vi "find_special_character_pairs.vi"(8 "error in (no error)":errorcluster, 10 "String Pair":T1={"Start Sting"="{", "End String"="}"}, 11 "Command String":string="TRIGger:AND:ENABle {{ON | 1} | {OFF | 0}}") -> (0 "error out":errorcluster, 2 "Pair Offset":cluster{"Start Offset":i32, "End offset":i32}[](array[cluster])=[{"Start Offset"=21, "End offset"=28}, {"Start Offset"=32, "End offset"=40}, {"Start Offset"=20, "End offset"=41}])   [LabVIEW 2018]
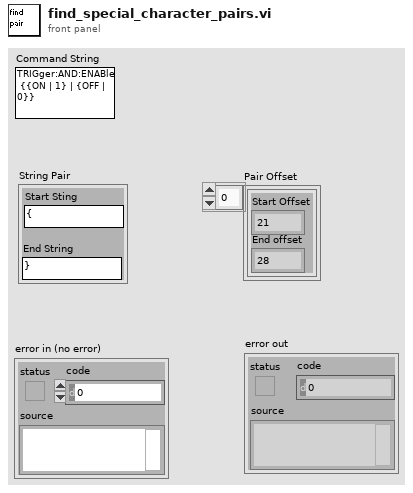
[diagram p1: front panel]
types:
  T1 = cluster{"Start Sting":string, "End String":string}
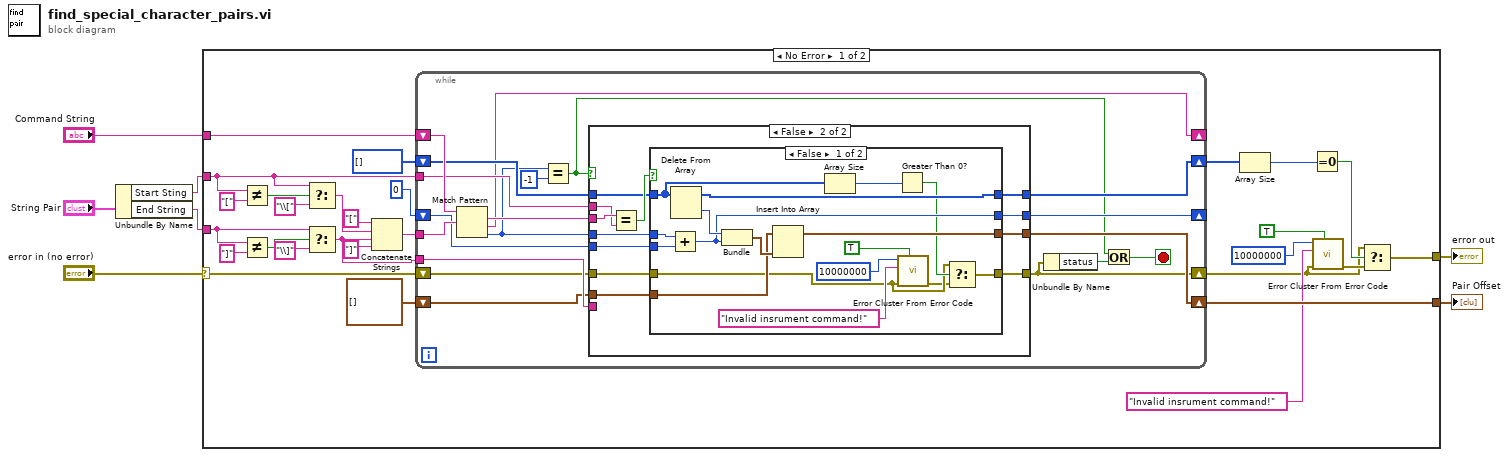
[diagram p0: block diagram]
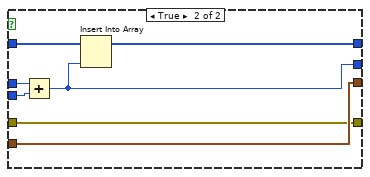
[diagram p3: hidden frame]
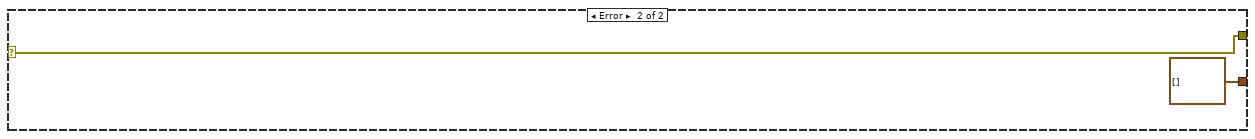
[diagram p4: hidden frame]
diagram:
  n1 = Unbundle By Name("String Pair") -> ("Start Sting"=w2:string, "End String"=w1:string)
  n2 = case shown="No Error" "error in (no error)" {
    selector: "error in (no error)" -> [w27 w96]
    tunnel: "Command String" -> [w33 _]
    tunnel: w1 -> [w10 _]
    tunnel: w2 -> [w8 _]
    tunnel: [w28 cluster{"Start Offset":i32, "End offset":i32}[] [] ("Pair Offset")] -> w6
    tunnel: [w18 w96] -> w4
    frame No Error {
      n3 = Not Equal?(x=w8, y="[") -> (x != y?=w15:bool)
      n4 = Not Equal?(x=w10, y="]") -> (x != y?=w12:bool)
      n5 = Select(t=w8, s=w15, f="\\[") -> (s? t:f=w13:string)
      n6 = Select(t=w10, s=w12, f="\\]") -> (s? t:f=w9:string)
      n7 = Concatenate Strings("[" ("string"), w13, w9, "]" ("string")) -> (w30:string)
      n8 = while {
        shift-right: [w41] -> _
        shift-left: w33 -> [w54]
        shift-right: [w45] -> _
        shift-left: 0 ("y") -> [w46]
        shift-right: [w44] -> w26
        shift-left: i32[] [] -> [w48]
        tunnel: w9 -> [w50]
        tunnel: w8 -> [w51]
        tunnel: w30 -> [w53]
        shift-right: [w42] -> w28
        shift-left: cluster{"Start Offset":i32, "End offset":i32}[] [] ("Pair Offset") -> [w43]
        shift-right: [w36] -> w19
        shift-left: w27 -> [w37]
        stop <- w38 stop-if-true
        n9 = Match Pattern(string=w54, regular expression=w53) -> (match substring=w49:string, after substring=w41:string, offset past match=w47:i32)  [unwired: 2 out]
        n10 = Equal?(x=w47, y=-1) -> (x = y?=w40:bool)
        n11 = case shown="False" w40 {
          tunnel: w51 -> [_ w69]
          tunnel: w50 -> [_ _]
          tunnel: w49 -> [_ w70]
          tunnel: w48 -> [w57 w67]
          tunnel: w47 -> [_ w66]
          tunnel: w46 -> [w58 w65]
          tunnel: [w58 w64] -> w45
          tunnel: [w57 w63] -> w44
          tunnel: w43 -> [w56 w62]
          tunnel: [w56 w61] -> w42
          tunnel: w37 -> [w55 w60]
          tunnel: [w55 w59] -> w36
          frame True {
          }
          frame False {
            n12 = Equal?(x=w70, y=w69) -> (x = y?=w68:bool)
            n13 = case shown="False" w68 {
              tunnel: w67 -> [w79 w92]
              tunnel: w66 -> [w87 w94]
              tunnel: w65 -> [w86 w93]
              tunnel: [w80 w91] -> w64
              tunnel: [w85 w90] -> w63
              tunnel: w62 -> [w83 w89]
              tunnel: [w82 w89] -> w61
              tunnel: w60 -> [w72 w88]
              tunnel: [w76 w88] -> w59
              frame False {
                n14 = Add(x=w87, y=w86) -> (x+y=w80:i32)
                n15 = Delete From Array(array=w79) -> (deleted portion=w81:i32, array with subset deleted=w85:i32[])  [unwired: 2 in]
                n16 = Bundle(w81, w80) -> (w84:cluster{i32, i32})  [unwired: 1 out]
                n17 = Insert Into Array(array=w83, new element=w84) -> (w82:cluster{"Start Offset":i32, "End offset":i32}[])  [unwired: 1 in]
                n18 = Array Size(array=w79) -> (size(s)=w78:i32)
                n19 = Greater Than 0?(x=w78) -> (x > 0?=w77:bool)
                n20 = call <vilib>:"Error Cluster From Error Code.vi"("show call chain? (False)"=TRUE, "error in (no error)"=w72, "error message (\"\")"="Invalid insrument command!" ("source"), "error code (0)"=10000000 ("code")) -> ("error out"=w71:errorcluster)  [unwired: 5 out]
                n21 = Select(t=w72, s=w77, f=w71) -> (s? t:f=w76:errorcluster)
              }
              frame True {
                n22 = Add(x=w94, y=w93) -> (x+y=w91:i32)
                n23 = Insert Into Array(array=w92, new element=w91) -> (w90:i32[])  [unwired: 1 in]
              }
            }
          }
        }
        n24 = Unbundle By Name(w36) -> ("status"=w39:bool)
        n25 = Or(x=w40, y=w39) -> (x .or. y?=w38:bool)
      }
      n26 = Array Size(array=w26) -> (size(s)=w25:i32)
      n27 = Equal To 0?(x=w25) -> (x = 0?=w24:bool)
      n28 = call <vilib>:"Error Cluster From Error Code.vi"("show call chain? (False)"=TRUE, "error in (no error)"=w19, "error message (\"\")"="Invalid insrument command!" ("source"), "error code (0)"=10000000 ("code")) -> ("error out"=w20:errorcluster)  [unwired: 5 out]
      n29 = Select(t=w19, s=w24, f=w20) -> (s? t:f=w18:errorcluster)
    }
    frame Error {
    }
  }
  "Pair Offset" <- w6
  "error out" <- w4
